vi "PH_ImageOperator.PC Write PSDB.vi"(0 "i ref in":refnum<vi>, 5 "error IO":errorcluster) -> (14 "i ref out":refnum<vi>, 19 "error out":errorcluster)   [LabVIEW 2014, in "PH_ImageOperator.lvlib"]
doc: "This is the proc case which writes data to the PHELIX shot data base."
uses:
  PH_ImageOperator.lvlib
  PH_PSDBWriter/PH_PSDBWriter.lvlib
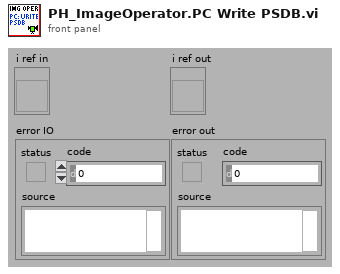
[diagram p1: front panel]
types:
  T1 = typedef "PH_PSDBWriter.lvlib/PH_PSDBWriter.Image dataset.ctl" = cluster{"name":string, "data":T2, "unit":string}
  T2 = typedef "IMAQ Image.ctl" = refnum<image>
  T3 = typedef "PH_PSDBWriter.lvlib/PH_PSDBWriter.Boolean dataset.ctl" = cluster{"name":string, "data":bool, "unit":string}
  T4 = typedef "PH_PSDBWriter.lvlib/PH_PSDBWriter.Numeric dataset.ctl" = cluster{"name":string, "data":dbl, "unit":string}
  T5 = typedef "PH_PSDBWriter.lvlib/PH_PSDBWriter.String dataset.ctl" = cluster{"name":string, "data":string, "unit":string}
  T6 = typedef "PH_PSDBWriter.lvlib/PH_PSDBWriter.2D dataset.ctl" = cluster{"name":string, "data":dbl[][], "axis description":T7}
  T7 = typedef "PSDB.lvlib/PSDB_AxisDescription.ctl" = cluster{"x axis label":string, "y axis label":string, "x axis unit":string, "y axis unit":string}
  T8 = typedef "PH_PSDBWriter.lvlib/PH_PSDBWriter.PSDB Dataset.ctl" = cluster{"Version":i32, "2D data Input":T6[], "Boolean Input":T3[], "Image Input":T1[], "Numeric Input":T4[], "String Input":T5[]}
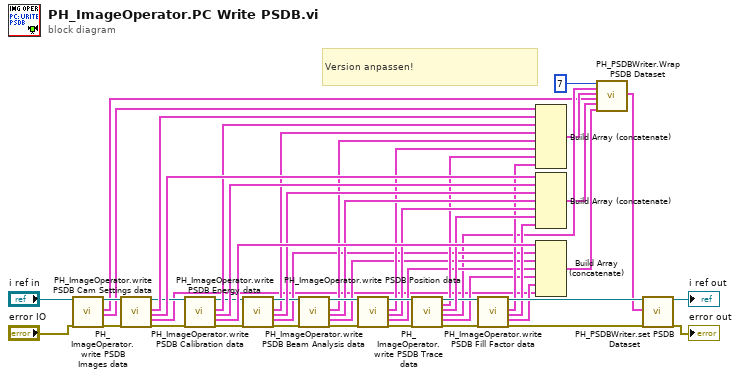
[diagram p0: block diagram]
diagram:
  # "Version anpassen!"
  n1 = call "PH_ImageOperator.write PSDB Images data.vi"("i ref in"="i ref in", "error in"="error IO") -> ("i ref out"=w49:refnum<vi>, "Images Image data"=w3:T1[], "Images Boolean data"=w42:T3[], "error out"=w48:errorcluster)  [unwired: 14 in]
  n2 = call "PH_ImageOperator.write PSDB Cam Settings data.vi"("i ref in"=w49, "error in"=w48) -> ("i ref out"=w44:refnum<vi>, "Cam Settings Boolean data"=w47:T3[], "Cam Settings Numeric data"=w46:T4[], "Cam Settings String data"=w1:T5[], "error out"=w45:errorcluster)  [unwired: 13 in]
  n3 = call "PH_ImageOperator.write PSDB Calibration data.vi"("i ref in"=w44, "error in"=w45) -> ("i ref out"=w39:refnum<vi>, "Calibration Boolean data"=w41:T3[], "Calibration Numeric data"=w40:T4[], "Calibration String data"=w43:T5[], "error out"=w38:errorcluster)  [unwired: 13 in]
  n4 = call "PH_ImageOperator.write PSDB Energy data.vi"("i ref in"=w39, "error in"=w38) -> ("i ref out"=w32:refnum<vi>, "Energy Boolean data"=w18:T3[], "Energy Numeric data"=w37:T4[], "Energy String data"=w12:T5[], "error out"=w30:errorcluster)  [unwired: 13 in]
  n5 = call "PH_ImageOperator.write PSDB Beam Analysis data.vi"("i ref in"=w32, "error in"=w30) -> ("i ref out"=w31:refnum<vi>, "BA Boolean data"=w28:T3[], "BA Numeric data"=w26:T4[], "BA String data"=w13:T5[], "error out"=w29:errorcluster)  [unwired: 13 in]
  n6 = call "PH_ImageOperator.write PSDB Position data.vi"("i ref in"=w31, "error in"=w29) -> ("i ref out"=w36:refnum<vi>, "Position Boolean data"=w16:T3[], "Position Numeric data"=w27:T4[], "Position String data"=w15:T5[], "error out"=w35:errorcluster)  [unwired: 13 in]
  n7 = call "PH_ImageOperator.write PSDB Trace data.vi"("i ref in"=w36, "error in"=w35) -> ("i ref out"=w24:refnum<vi>, "Trace Boolean data"=w17:T3[], "Trace Numeric data"=w25:T4[], "Trace 2D data"=w6:T6[], "Trace String data"=w14:T5[], "error out"=w22:errorcluster)  [unwired: 12 in]
  n8 = call "PH_ImageOperator.write PSDB Fill Factor data.vi"("i ref in"=w24, "error in"=w22) -> ("i ref out"=w23:refnum<vi>, "Fill Factor Boolean data"=w20:T3[], "Fill Factor Numeric data"=w19:T4[], "Fill Factor String data"=w21:T5[], "error out"=w10:errorcluster)  [unwired: 13 in]
  n9 = Build Array (concatenate)(w42, w47, w41, w18, w28, w16, w17, w20) -> (w4:T3[])
  n10 = Build Array (concatenate)(w46, w40, w37, w26, w27, w25, w19) -> (w5:T4[])
  n11 = Build Array (concatenate)(w43, w12, w13, w15, w14, w21, w1) -> (w7:T5[])
  n12 = call "PH_PSDBWriter.Wrap PSDB Dataset.vi"("Version"=7, "2D data Input"=w6, "Boolean Input"=w4, "Image Input"=w3, "Numeric Input"=w5, "String Input"=w7) -> ("PSDB Dataset"=w8:T8)  [unwired: 13 in]
  n13 = call "PH_PSDBWriter.set PSDB Dataset.vi"("VI in"=w23, "PSDB Dataset"=w8, "error in (no error)"=w10) -> ("VI out"=→"i ref out":refnum<vi>, "error out"=→"error out":errorcluster)  [unwired: 15 in]
